vi "steerer split.vi"(1 "Steerer in":dbl format="%#_4g") -> (6 "Steerer +":dbl format="%#_4g", 7 "Steerer -":dbl format="%#_4g")   [LabVIEW 2016, in "Low energy.lvlib"]
doc: "This vi takes the set value for a steerer and splits it to a positive and negative signal"
uses:
  Low energy.lvlib
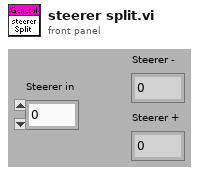
[diagram p1: front panel]
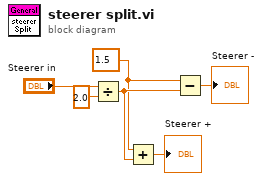
[diagram p0: block diagram]
diagram:
  w3 = 1.5 ("x")
  n1 = Divide(x="Steerer in", y=2.0) -> (x/y=w4:dbl)
  n2 = Add(x=w3, y=w4) -> (x+y=→"Steerer +":dbl)
  n3 = Subtract(x=w3, y=w4) -> (x-y=→"Steerer -":dbl)
